vi "Split.vi"(6 "delimiter":string, 11 "String":string) -> (3 "Array Result":string[](array[string]))   [LabVIEW 2013]
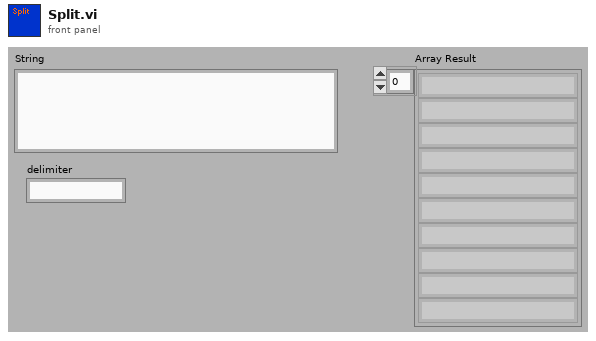
[diagram p1: front panel]
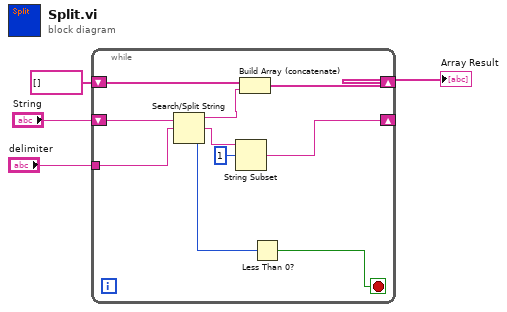
[diagram p0: block diagram]
diagram:
  n1 = while {
    shift-right: [w8] -> _
    shift-left: "String" -> [w14]
    shift-right: [w11] -> w2
    shift-left: string[] [] -> [w12]
    tunnel: "delimiter" -> [w5]
    stop <- w6 stop-if-true
    n2 = Search/Split String(string=w14, search string/char (-)=w5) -> (substring before match=w13:string, match + rest of string=w10:string, offset of match=w7:i32)  [unwired: 1 out]
    n3 = String Subset(string=w10, offset (0)=1) -> (substring=w8:string)  [unwired: 1 out]
    n4 = Build Array (concatenate)(w12, w13) -> (w11:string[])
    n5 = Less Than 0?(x=w7) -> (x < 0?=w6:bool)
  }
  "Array Result" <- w2
